vi "Vision Processing.vi"(8 "error in (no error)":errorcluster, 11 "Image Size":T1=enum."320x240") -> ()   [LabVIEW 2017]
uses:
  Vision Support Code/Camera Types.ctl
  <vilib>/Rock Robotics/WPI/Camera/WPI_CameraImageSize.ctl
  <vilib>/Rock Robotics/WPI/Camera/WPI_CameraWhite Balance Values.ctl
  <vilib>/Rock Robotics/WPI/Camera/WPI_CameraExposure Values.ctl
  <vilib>/Rock Robotics/WPI/Camera/WPI_CameraFrameRate.ctl
  <vilib>/Rock Robotics/SystemInterfaces/DIO/FPGA_DIOPWMChannel.ctl
  <vilib>/Rock Robotics/SystemInterfaces/DIO/FPGA_DIOChannel.ctl
  <vilib>/Rock Robotics/WPI/MotorControl/WPI_MotorControlOpen NidecBrushless.vi
  Robot Global Data.vi
  <vilib>/Rock Robotics/Network Tables/NT Write Number.vi
  <vilib>/vision/NI_Vision_Development_Module.lvlib
panel:
  out "normalized":dbl
  in  "Min Component %":dbl=15.0
  out "loop ms":u32
  in  "Display Original":bool
  in  "Display Mask":bool
  out "Instructions:":string="Connect a USB or IP camera to your roboRIO. If using a ring light and retroreflective tape, use Camera Settings outside the loop create a dark image with bright and colorful stripes. If used wihtout a ring light, brighten the images so that stripes are visible.\n\nLED Color can encoded as HSL or related color modes. Calibrate to the same color as the strips being reflected to the camera. Unlike the desktop example, this LED color must be set by hand. You can also put the calibration on the dashboard and send the LED Color to the RT code using Network Tables.\n\nThe Display buttons affects whether images are displayed on the panel. It takes quite a bit of CPU  to compress and transmit the images for display.\n\nAdjust Score Cutoff to make the code more or less picky. If the color is not very unique, you may need to increase the number of particles considered. The diagram uses a Size Limit to ignore colored things that are too small. You may need to adjust it if you are targetting from far away.\n\nResults give you the distance to the target, the center and box in a normalized (-1 to 1) and pixel coordinates.\n\nBe sure to read about setting camera exposure and brightness to help simplify your image and acquire color saturated images.\n\nThere are lots of comments on the diagram to explain the code."
  in  "Color Mode":u16(ring)=2 items=["RGB", "HSL", "HSV", "HSI"]
  in  "Particles":dbl=5.0
  in  "Score Cutoff %":dbl=75.0
  in  "Camera Type":T2=enum."MS HD3000 square"
  out "Result":T3 {"Score" format="%#_3g"; "Pixels"."Rectangle"."Numeric 5" format="%#_3g"; "Pixels"."Rectangle"."Numeric 3" format="%#_3g"; "Pixels"."Rectangle"."Numeric 2" format="%#_3g"; "Pixels"."Rectangle"."Numeric" format="%#_3g"; "Normalized"."Rectangle"."Numeric 5" format="%#_2g"; "Normalized"."Rectangle"."Numeric 3" format="%#_2g"; "Normalized"."Rectangle"."Numeric 2" format="%#_2g"; "Normalized"."Rectangle"."Numeric" format="%#_2g"; "Normalized"."Center"."?" format="%#_3g"; "Normalized"."Center"."?" format="%#_3g"; "Distance (ft)" format="%#_3g"}
  out "Qualified Particles":i32
  in  "LED Color":T4={"Hue"={107.81818389892578, 139.81818389892578}, "Sat"={176.07142857142858, 255.0}, "Val"={40.53571428571429, 255.0}} {"Hue" scale=0.0..255.0 scale format="%#_3g"}
  out "Mask":T5(plugin-control)
  out "Original Image":T5(plugin-control)
  # "Good target, distance ft"
  # "Bad target"
  # "Score in %"
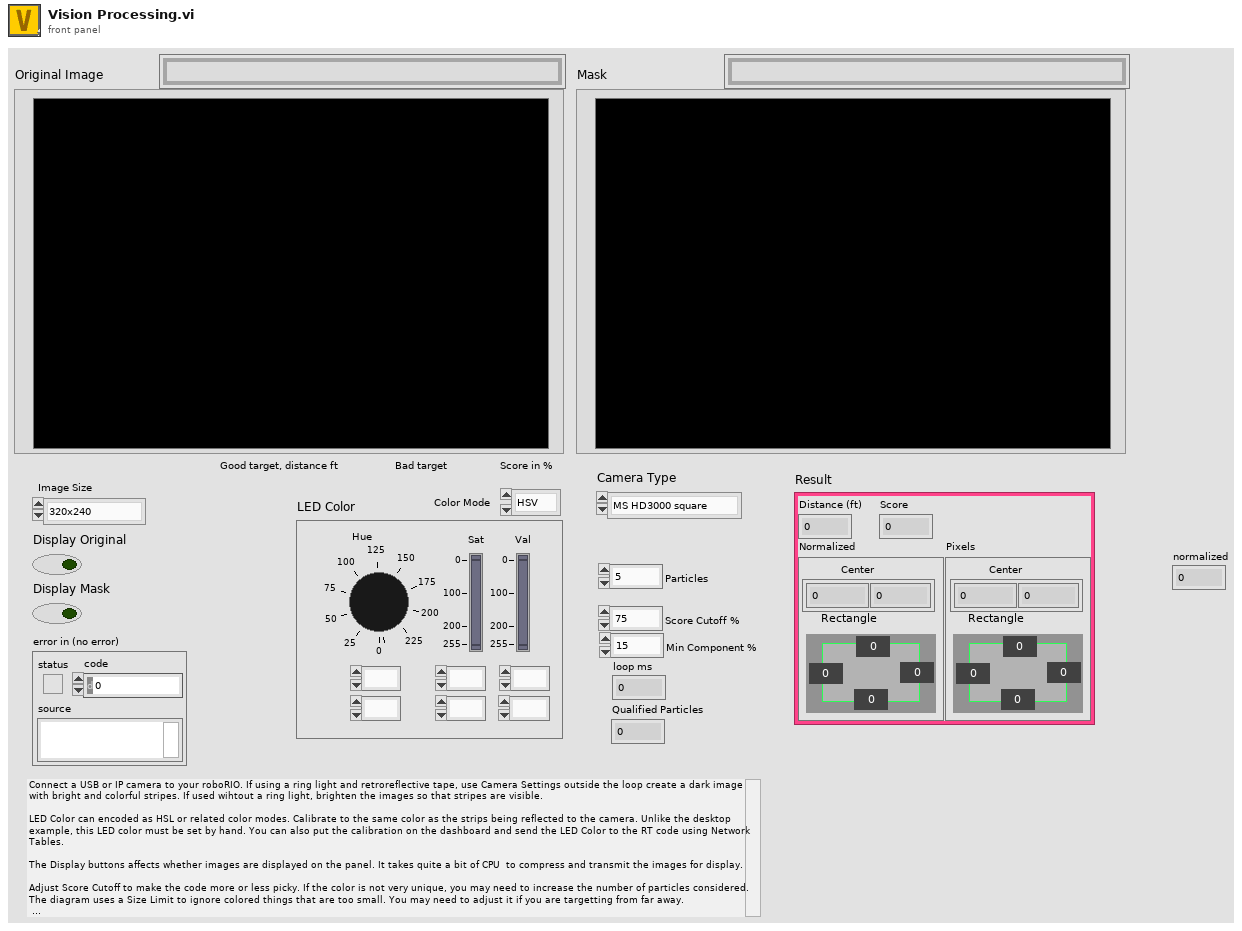
[diagram p1: front panel]
types:
  T1 = typedef "WPI_CameraImageSize.ctl" = enum16{"640x480", "320x240", "160x120", "Custom"}
  T2 = typedef "Camera Types.ctl" = enum16{"206", "1011", "1013", "MS HD3000 square", "MS HD3000 640x480"}
  T3 = cluster{"Distance (ft)":dbl, "Score":dbl, "Normalized":cluster{"Center":cluster{dbl, dbl}, "Rectangle":cluster{"Numeric":dbl, "Numeric 2":dbl, "Numeric 3":dbl, "Numeric 5":dbl}}, "Pixels":cluster{"Center":cluster{dbl, dbl}, "Rectangle":cluster{"Numeric":dbl, "Numeric 2":dbl, "Numeric 3":dbl, "Numeric 5":dbl}}}
  T4 = cluster{"Hue":cluster{dbl, dbl}, "Sat":cluster{dbl, dbl}, "Val":cluster{dbl, dbl}}
  T5 = typedef "IMAQ Image.ctl" = refnum<image>
  T6 = typedef "FPGA_DIOChannel.ctl" = enum8{"DIO 0", "DIO 1", "DIO 2", "DIO 3", "DIO 4", "DIO 5", "DIO 6", "DIO 7", "DIO 8", "DIO 9", "DIO MXP 0", "DIO MXP 1", "DIO MXP 2", "DIO MXP 3", "DIO MXP 4", "DIO MXP 5", "DIO MXP 6", "DIO MXP 7", "DIO MXP 8", "DIO MXP 9", "DIO MXP 10", "DIO MXP 11", "DIO MXP 12", "DIO MXP 13", "DIO MXP 14", "DIO MXP 15", "SPI Port CS1", "SPI Port CS2", "SPI Port CS3", "SPI Port MISO", "SPI Port MOSI", "Invalid"}
  T7 = typedef "FPGA_DIOPWMChannel.ctl" = enum8{"PWM 0", "PWM 1", "PWM 2", "PWM 3", "PWM 4", "PWM 5", "PWM 6", "PWM 7", "PWM 8", "PWM 9", "PWM MXP 0", "PWM MXP 1", "PWM MXP 2", "PWM MXP 3", "PWM MXP 4", "PWM MXP 5", "PWM MXP 6", "PWM MXP 7", "PWM MXP 8", "PWM MXP 9", "Invalid"}
  T8 = typedef "WPI_CameraFrameRate.ctl" = u32
  T9 = typedef "WPI_CameraExposure Values.ctl" = enum16{"Auto", "Flicker-free 50 Hz", "Flicker-free 60 Hz", "Hold current", "Custom"}
  T10 = typedef "WPI_CameraWhite Balance Values.ctl" = enum16{"Auto", "Fixed indoor", "Fixed outdoor 1", "Fixed outdoor 2", "Fixed fluorescent 1", "Fixed fluorescent 2", "Hold current", "Custom"}
  T11 = typedef "Particle Parameters" = i32
  T12 = typedef "Image Type" = u32
  T13 = typedef "WPI_MotorControlDeviceRef.ctl" = cluster{"DeviceStatus":errorcluster, "Type":T14, "PWM":cluster{"PWM Channel":T7, "DeadBand":T15}, "CAN":cluster{"Device Number":u8, "SetOutput VI Ref":variant, "GetOutput VI Ref":variant, "Enable VI Ref":variant, "Disable VI Ref":variant, "Data":variant}, "Invert":bool, "DIO PWM":cluster{"PWM \"Enable\" Channel":T7, "DIOChannel":T6, "PWM Rate":dbl}}
  T14 = typedef "WPI_MotorControlType.ctl" = enum16{"PWM", "CAN", "DIO PWM"}
  T15 = typedef "WPI_PWMDeadband.ctl" = cluster{"Name":string, "maxPositivePwm":i32, "minPositivePwm":i32, "centerPwm":i32, "maxNegativePwm":i32, "minNegativePwm":i32, "angularRange":u16}
  T16 = typedef "WPI_CameraDevRef.ctl" = cluster{"Camera Address":string, "CameraStatus":errorcluster}
  T17 = cluster{"Score":dbl, "Rect":cluster{"Left":dbl, "Top":dbl, "Right":dbl, "Bottom":dbl}, "Full Scores":cluster{"Aspect Ratio":dbl, "Top Position":dbl, "Bottom Position":dbl, "Left Gap":dbl, "Width":dbl, "Height Ratio":dbl}}[]
  T18 = cluster{"Score":dbl, "Rect":cluster{"Left":dbl, "Top":dbl, "Right":dbl, "Bottom":dbl}, "Full Scores":cluster{"Aspect Ratio":dbl, "Top Position":dbl, "Bottom Position":dbl, "Left Gap":dbl, "Width":dbl, "Height Ratio":dbl}}
  T19 = cluster{"Left":dbl, "Top":dbl, "Right":dbl, "Bottom":dbl}
  T20 = cluster{"Center":cluster{dbl, dbl}, "Rectangle":cluster{"Numeric":dbl, "Numeric 2":dbl, "Numeric 3":dbl, "Numeric 5":dbl}}
  T21 = cluster{"Numeric":dbl, "Numeric 2":dbl, "Numeric 3":dbl, "Numeric 5":dbl}
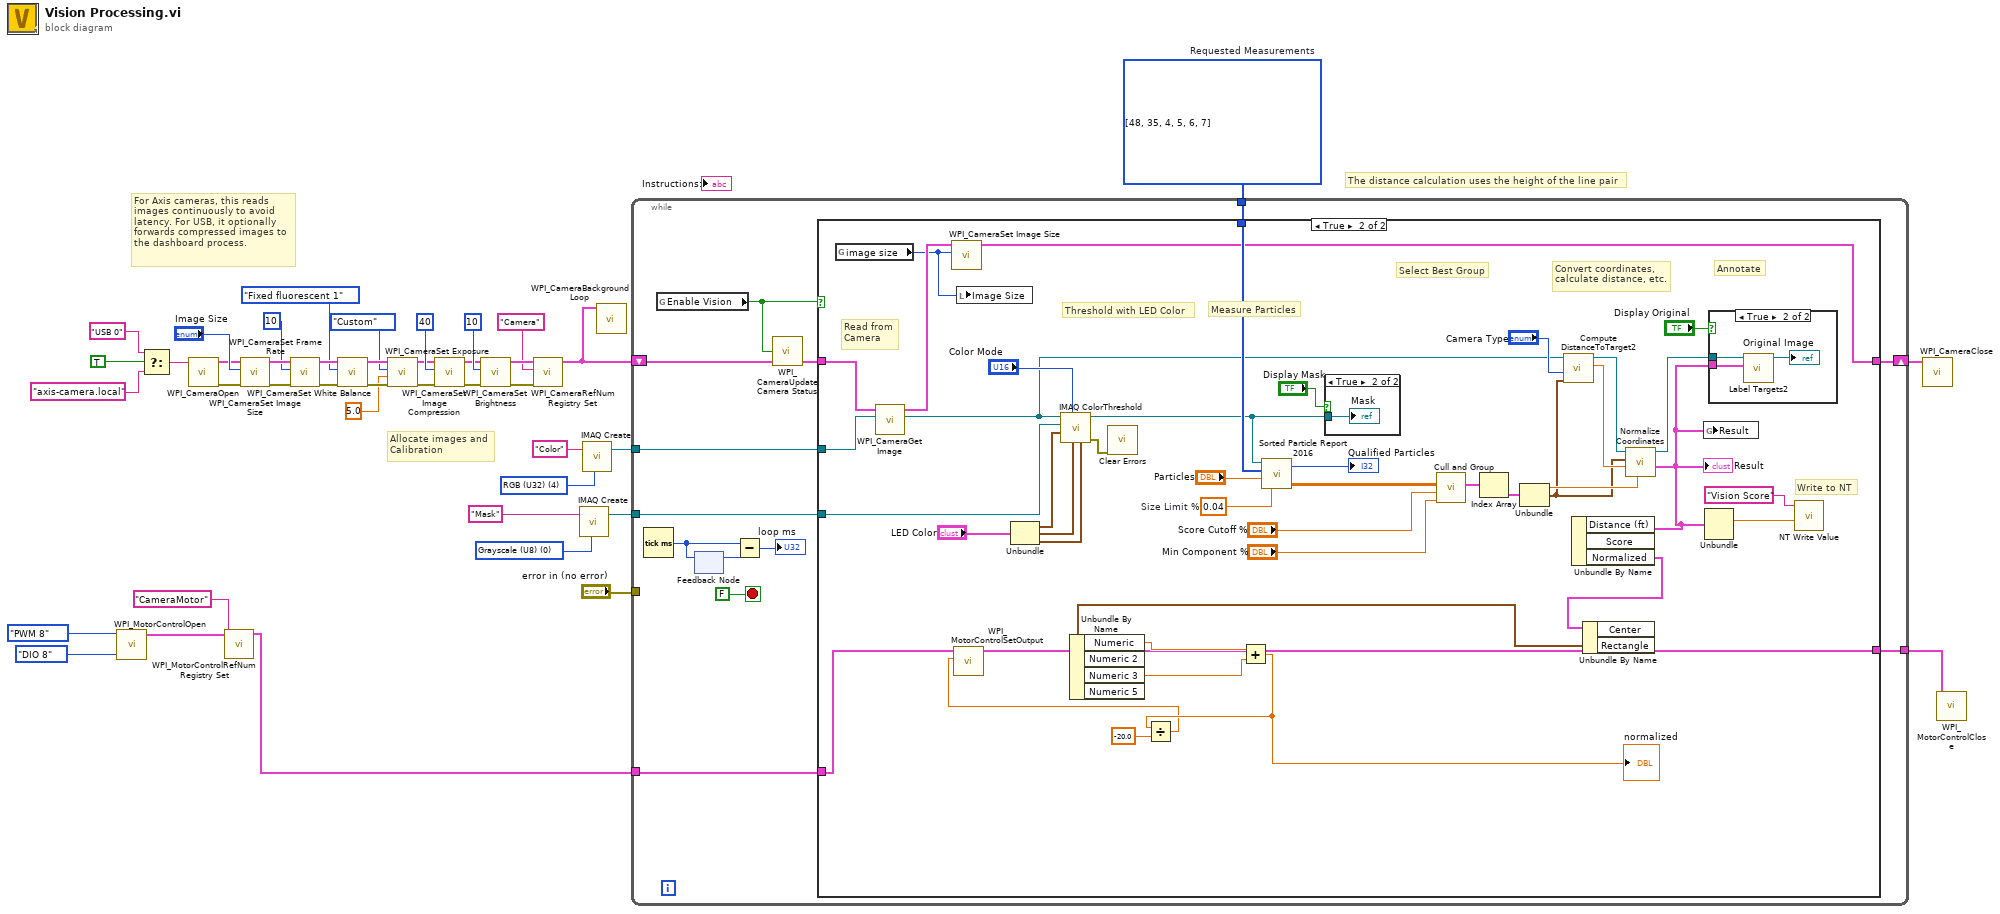
[diagram p0: block diagram]
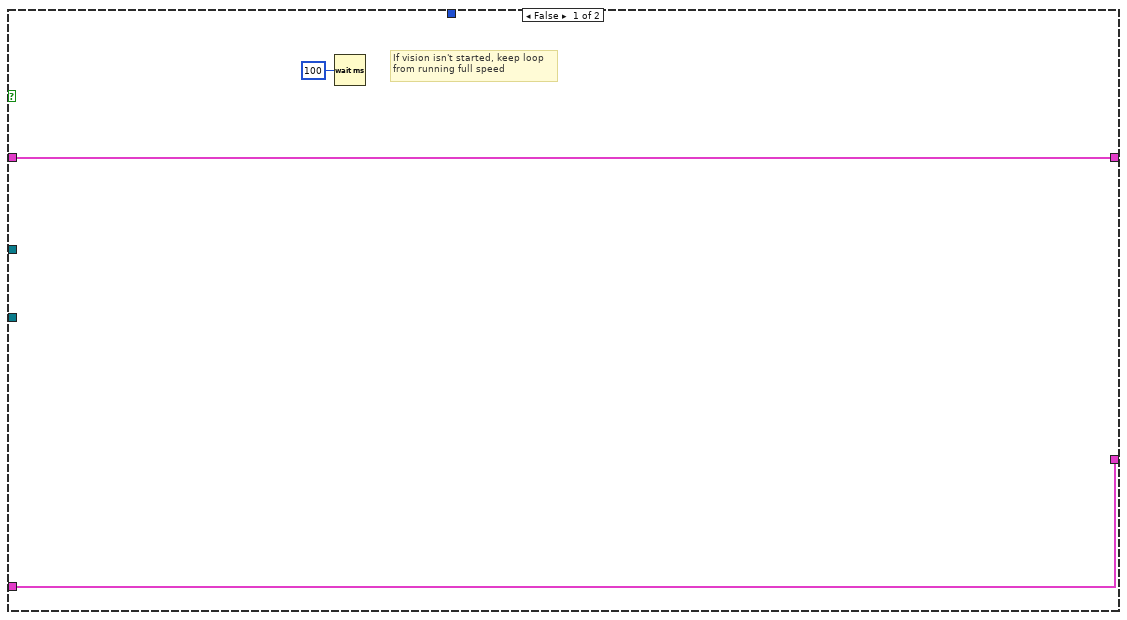
[diagram p2: hidden frame]
diagram:
  w37 = T11[] [48, 35, 4, 5, 6, 7] items=["Center of Mass X", "Center of Mass Y", "First Pixel X", "First Pixel Y", "Bounding Rect Left", "Bounding Rect Top", "Bounding Rect Right", "Bounding Rect Bottom", "Max Feret Diameter Start X", "Max Feret Diameter Start Y", "Max Feret Diameter End X", "Max Feret Diameter End Y", "Max Horiz. Segment Length Left", "Max Horiz. Segment Length Right", "Max Horiz. Segment Length Row", "-", "Bounding Rect Width", "Bounding Rect Height", "Bounding Rect Diagonal", "Perimeter", "Convex Hull Perimeter", "Holes' Perimeter", "Max Feret Diameter", "Equivalent Ellipse Major Axis", "Equivalent Ellipse Minor Axis", "Equivalent Ellipse Minor Axis (Feret)", "Equivalent Rect Long Side", "Equivalent Rect Short Side", "Equivalent Rect Diagonal", "Equivalent Rect Short Side (Feret)", "Average Horiz. Segment Length", "Average Vert. Segment Length", "Hydraulic Radius", "Waddel Disk Diameter", "-", "Area", "Holes' Area", "Particle & Holes' Area", "Convex Hull Area", "Image Area", "-", "Number of Holes", "Number of Horiz. Segments", "Number of Vert. Segments", "-", "Orientation", "Max Feret Diameter Orientation", "-", "% Area/Image Area", "% Area/(Particle & Holes' Area)", "Ratio of Equivalent Ellipse Axes", "Ratio of Equivalent Rect Sides", "-", "Elongation Factor", "Compactness Factor", "Heywood Circularity Factor", "Type Factor", "-", "Sum X", "Sum Y", "Sum XX", "Sum XY", "Sum YY", "Sum XXX", "Sum XXY", "Sum XYY", "Sum YYY", "-", "Moment of Inertia XX", "Moment of Inertia XY", "Moment of Inertia YY", "Moment of Inertia XXX", "Moment of Inertia XXY", "Moment of Inertia XYY", "Moment of Inertia YYY", "Norm. Moment of Inertia XX", "Norm. Moment of Inertia XY", "Norm. Moment of Inertia YY", "Norm. Moment of Inertia XXX", "Norm. Moment of Inertia XXY", "Norm. Moment of Inertia XYY", "Norm. Moment of Inertia YYY", "Hu Moment 1", "Hu Moment 2", "Hu Moment 3", "Hu Moment 4", "Hu Moment 5", "Hu Moment 6", "Hu Moment 7"]  # Requested Measurements
  w40 = T12 0 items=["Grayscale (U8)", "Grayscale (I16)", "Grayscale (SGL)", "Complex (CSG)", "RGB (U32)", "HSL (U32)", "RGB (U64)", "Grayscale (U16)"] ("Image Type")
  w41 = T12 4 items=["Grayscale (U8)", "Grayscale (I16)", "Grayscale (SGL)", "Complex (CSG)", "RGB (U32)", "HSL (U32)", "RGB (U64)", "Grayscale (U16)"] ("Image Type")
  # "For Axis cameras, this reads\nimages continuously to avoid\nlatency. For USB, it optionally\nforwards compressed images to\nthe dashboard process."
  # "The distance calculation uses the height of the line pair"
  # "Allocate images and\nCalibration"
  n1 = call-poly <vilib>:"WPI_MotorControlOpen.vi"("DIOChannel"=FPGA_DIOChannel."DIO 8" ("DIO Channel"), "PWM Channel"=FPGA_DIOPWMChannel."PWM 8") -> ("MotorControlDeviceRef"=w6:T13)  [unwired: 8 in, 1 out]
  n2 = Select(t="USB 0" ("format string"), s=TRUE ("dot notation? (F)"), f="axis-camera.local" ("format string")) -> (s? t:f=w11:string)
  n3 = call <vilib>:"WPI_CameraOpen.vi"("Camera Address"=w11) -> ("error out"=w23:errorcluster, "CameraDevRef"=w24:T16)  [unwired: 1 in, 8 out]
  n4 = call <vilib>:"WPI_MotorControlRefNum Registry Set.vi"("refnum name"="CameraMotor", "MotorControlDevRef"=w6) -> ("MotorControlDevRef"=w2:T13)  [unwired: 8 in, 1 out]
  n5 = call <vilib>:"WPI_CameraSet Image Size.vi"("error in (no error)"=w23, "Image Size"="Image Size", "CameraDevRef"=w24) -> ("error out"=w22:errorcluster, "CameraDevRef Out"=w25:T16)  [unwired: 1 in, 6 out]
  n6 = call <vilib>:"WPI_CameraSet Frame Rate.vi"("error in (no error)"=w22, "Frame Rate (fps)"=T8 10, "CameraDevRef"=w25) -> ("error out"=w21:errorcluster, "CameraDevRef Out"=w27:T16)  [unwired: 7 out]
  n7 = call <vilib>:"WPI_CameraSet White Balance.vi"("error in (no error)"=w21, "White Balance"=WPI_CameraWhite_Balance_Values."Fixed fluorescent 1", "CameraDevRef"=w27) -> ("error out"=w20:errorcluster, "CameraDevRef Out"=w26:T16)  [unwired: 1 in, 6 out]
  n8 = call <vilib>:"WPI_CameraSet Exposure.vi"("error in (no error)"=w20, "Exposure (%)"=5.0, "Exposure"=WPI_CameraExposure_Values."Custom", "CameraDevRef"=w26) -> ("error out"=w19:errorcluster, "CameraDevRef Out"=w29:T16)  [unwired: 6 out]
  n9 = call <vilib>:"WPI_CameraSet Image Compression.vi"("error in (no error)"=w19, "Compression"=40, "CameraDevRef"=w29) -> ("error out"=w18:errorcluster, "CameraDevRef Out"=w28:T16)  [unwired: 7 out]
  n10 = call <vilib>:"WPI_CameraSet Brightness.vi"("error in (no error)"=w18, "Brightness"=10, "CameraDevRef"=w28) -> ("error out"=w17:errorcluster, "CameraDevRef Out"=w35:T16)  [unwired: 1 in, 6 out]
  n11 = call <vilib>:"WPI_CameraRefNum Registry Set.vi"("error in (no error)"=w17, "refnum name"="Camera", "CameraDevRef"=w35) -> ("CameraDevRef"=w10:T16)  [unwired: 1 in, 7 out]
  n12 = call "IMAQ Create"("Image Name"="Mask", "Image Type"=w40) -> ("New Image"=w38:T5)  [unwired: 2 in, 2 out]
  n13 = call "IMAQ Create"("Image Name"="Color", "Image Type"=w41) -> ("New Image"=w36:T5)  [unwired: 2 in, 2 out]
  n14 = call <vilib>:"WPI_CameraBackground Loop.vi"("CameraDevRef"=w10) -> ()  [unwired: 11 in]
  n15 = while {
    tunnel: w36 -> [w52]
    tunnel: w38 -> [w54]
    tunnel: w37 -> [w53]
    shift-right: [w51] -> w9
    shift-left: w10 -> [w50]
    tunnel: "error in (no error)" -> [_]
    tunnel: w2 -> [w44]
    tunnel: [w43] -> w1
    stop <- FALSE stop-if-true
    n16 = Tick Count (ms)() -> (millisecond timer value=w46:u32)
    n17 = global read "Robot Global Data.vi" "Enable Vision"() -> (w48:bool)
    n18 = feedback-in #1(w46) -> ()
    n19 = feedback #1() -> (w47:u32)  [unwired: 1 in]
    n20 = Subtract(x=w46, y=w47) -> (x-y=→"loop ms":u32)
    n21 = call <vilib>:"WPI_CameraUpdate Camera Status.vi"("CameraDevRef In"=w50, "Enable Vision"=w48) -> ("CameraDevRef Out"=w49:T16)  [unwired: 3 in]
    n22 = case shown="True" w48 {
      tunnel: w54 -> [_ w101]
      tunnel: w53 -> [_ w97]
      tunnel: w49 -> [w58 w83]
      tunnel: w52 -> [_ w82]
      tunnel: [w58 w77] -> w51
      tunnel: w44 -> [w56 w63]
      tunnel: [w56 w60] -> w43
      frame False {
        # "If vision isn't started, keep loop\nfrom running full speed"
        n23 = Wait (ms)(milliseconds to wait=u32 100) -> ()  [unwired: 1 out]
      }
      frame True {
        w95 = 0.04  # Size Limit %
        # "Write to NT"
        # "Read from\nCamera"
        # "Measure Particles"
        # "Convert coordinates,\ncalculate distance, etc."
        # "Annotate"
        # "Select Best Group"
        # "Threshold with LED Color"
        n24 = global read "Robot Global Data.vi" "image size"() -> (w76:T1)
        n25 = call <vilib>:"WPI_CameraGet Image.vi"("Image"=w82, "CameraDevRef"=w83) -> ("Image Out"=w81:T5, "CameraDevRef Out"=w78:T16)  [unwired: 7 in, 1 out]
        n26 = call <vilib>:"WPI_CameraSet Image Size.vi"("Image Size"=w76, "CameraDevRef"=w78) -> ("CameraDevRef Out"=w77:T16)  [unwired: 2 in, 7 out]
        n27 = local write "Image Size"(w76) -> ()
        n28 = Unbundle("LED Color") -> ("Hue"=w100:cluster{dbl, dbl}, "Sat"=w99:cluster{dbl, dbl}, "Val"=w98:cluster{dbl, dbl})
        n29 = call "IMAQ ColorThreshold"("Blue or Luma or Val or Inten Range"=w98, "Green or Sat Range"=w99, "Color Mode"="Color Mode", "Red or Hue Range"=w100, "Image Dst"=w101, "Image Src"=w81) -> ("error out"=w94:errorcluster, "Image Dst Out"=w90:T5)  [unwired: 4 in]
        n30 = call <vilib>:"Clear Errors.vi"("error in (no error)"=w94) -> ()  [unwired: 5 in, 2 out]
        n31 = call "Sorted Particle Report 2016.vi"("Min Area Size %"=w95, "Particle Count Limit"="Particles", "Pixel Measurements"=w97, "Image in"=w90) -> ("Sorted Data"=w92:dbl[][], "Particles"=→"Qualified Particles":i32)
        n32 = case shown="True" "Display Mask" {
          tunnel: w90 -> [_ w105]
          frame False {
          }
          frame True {
            "Mask" <- w105
          }
        }
        n33 = call "Cull and Group.vi"("Min Compnt %"="Min Component %", "Score Cutoff %"="Score Cutoff %", "Sorted Data"=w92) -> ("Best Targets above cutoff"=w73:T17)  [unwired: 8 in]
        n34 = Index Array(array=w73) -> (element=w72:T18)  [unwired: 1 in]
        n35 = Unbundle(w72) -> ("Score"=w71:dbl, "Rect"=w70:T19)  [unwired: 1 out]
        n36 = call "Compute DistanceToTarget2.vi"("Rect"=w70, "Camera Type"="Camera Type", "Image Src"=w81) -> ("Distance (ft)"=w88:dbl, "Image Dst Out"=w87:T5)  [unwired: 7 in]
        n37 = call "Normalize Coordinates.vi"("Score"=w71, "Distance"=w88, "Bounding box"=w70, "Image in"=w87) -> ("Results"=w68:T3, "Image out"=w86:T5)  [unwired: 6 in]
        "Result" <- w68
        n38 = Unbundle By Name(w68) -> ("Normalized"=w67:T20)  [unwired: 2 out]
        n39 = Unbundle By Name(w67) -> ("Rectangle"=w66:T21)  [unwired: 1 out]
        n40 = Unbundle By Name(w66) -> ("Numeric"=w65:dbl, "Numeric 3"=w64:dbl)  [unwired: 2 out]
        n41 = Add(x=w65, y=w64) -> (x+y=w61:dbl)
        "normalized" <- w61
        n42 = Divide(x=w61, y=-20.0) -> (x/y=w59:dbl)
        n43 = call <vilib>:"WPI_MotorControlSetOutput.vi"("Output"=w59, "MotorControlDevRef"=w63) -> ("MotorControlDevRef"=w60:T13)  [unwired: 7 in, 2 out]
        n44 = global write "Robot Global Data.vi" "Result"(w68) -> ()
        n45 = Unbundle(w68) -> ("Score"=w75:dbl)  [unwired: 3 out]
        n46 = case shown="True" "Display Original" {
          tunnel: w86 -> [_ w103]
          tunnel: w68 -> [_ w102]
          frame False {
          }
          frame True {
            n47 = call "Label Targets2.vi"("Results"=w102, "Image in"=w103) -> ("Image out"=→"Original Image":T5)  [unwired: 9 in]
          }
        }
        n48 = call-poly <vilib>:"NT Write Value.vi"("Numeric"=w75, "Name"="Vision Score") -> ()  [unwired: 9 in, 1 out]
      }
    }
  }
  n49 = call <vilib>:"WPI_CameraClose.vi"("CameraDevRef"=w9) -> ()  [unwired: 1 in, 10 out]
  n50 = call <vilib>:"WPI_MotorControlClose.vi"("MotorControlDevRef"=w1) -> ()  [unwired: 10 in, 1 out]
